vi "Icon Initialization.vi"(7 "LabVIEW Icon in":string, 8 "error in (no error)":errorcluster, 11 "Data in":T1={"Class"={"Ants"=refnum, "Layer"=refnum, "Templates"=refnum, "Icon"=refnum, "Glyph"=refnum, "Settings"=refnum, "Tools"=refnum}, "Ref"={"Add Layer"=refnum, "Remove Layer"=refnum, "Line Text"=[], "Body Text Spec"=refnum, "DNL_Font"=refnum, "glyph path str"=refnum, "templates path str"=refnum, "Arrow Up"=refnum, "Arrow Down"=refnum, "IE VI Ref"=refnum, "Glyphs tree"=refnum, "Templates tree"=refnum, "Layer Icon Text"=refnum, "Layer Template"=refnum, "Clipboard"=refnum, "BW icon in"=refnum, "Color icon in"=refnum, "Layer Clust"=refnum, "Body Text"=refnum, "DNL_Framework Templates"=refnum, "Search Templates"=refnum, "TextMarker"=refnum, "Tab Control"=refnum, "Search Glyphs"=refnum, "Line Color"=refnum, "DNL_Glyphs []"=refnum, "Fill Color"=refnum, "Tools"=refnum, "Glyphs tree"=refnum, "Icon"=refnum, "Preview"=refnum, "Ants"=refnum, "Terminals"=refnum, "menu reference"=refnum, "LayerNames"=[], "GlyphLoadAnimation"=refnum, "TemplateLoadAnimation"=refnum, "refreshGlyphs"=refnum, "refreshTemplates"=refnum}, "Support"={"AntsRect"={"left"=0, "top"=0, "right"=0, "bottom"=0}, "Mouse Move Coords"={"Horizontal"=0, "Vertical"=0}, "Mouse Down Coords"={"Horizontal"=0, "Vertical"=0}, "Temp Coord"={"Horizontal"=0, "Vertical"=0}, "Action"=enum."Default", "Edge Color"=4914962, "Fill Color"=16860, "Mouse Down?"=FALSE, "Draft Mode?"=FALSE, "Temp Icon"=bytes[3102], "CTRL Pressed"=FALSE, "Move Selection?"=FALSE, "AntsRect Orig"={"left"=0, "top"=0, "right"=0, "bottom"=0}, "Text"="", "TM Set?"=FALSE, "Mouse inside icon?"=FALSE, "Tool (old value)"=0, "Pencil Move Color"=0, "Swap Colors?"=FALSE, "Shift pressed?"=FALSE}}) -> (0 "error out":errorcluster, 3 "Data out":T1={"Class"={"Ants"=refnum, "Layer"=refnum, "Templates"=refnum, "Icon"=refnum, "Glyph"=refnum, "Settings"=refnum, "Tools"=refnum}, "Ref"={"Add Layer"=refnum, "Remove Layer"=refnum, "Line Text"=[], "Body Text Spec"=refnum, "DNL_Font"=refnum, "glyph path str"=refnum, "templates path str"=refnum, "Arrow Up"=refnum, "Arrow Down"=refnum, "IE VI Ref"=refnum, "Glyphs tree"=refnum, "Templates tree"=refnum, "Layer Icon Text"=refnum, "Layer Template"=refnum, "Clipboard"=refnum, "BW icon in"=refnum, "Color icon in"=refnum, "Layer Clust"=refnum, "Body Text"=refnum, "DNL_Framework Templates"=refnum, "Search Templates"=refnum, "TextMarker"=refnum, "Tab Control"=refnum, "Search Glyphs"=refnum, "Line Color"=refnum, "DNL_Glyphs []"=refnum, "Fill Color"=refnum, "Tools"=refnum, "Glyphs tree"=refnum, "Icon"=refnum, "Preview"=refnum, "Ants"=refnum, "Terminals"=refnum, "menu reference"=refnum, "LayerNames"=[], "GlyphLoadAnimation"=refnum, "TemplateLoadAnimation"=refnum, "refreshGlyphs"=refnum, "refreshTemplates"=refnum}, "Support"={"AntsRect"={"left"=0, "top"=0, "right"=0, "bottom"=0}, "Mouse Move Coords"={"Horizontal"=0, "Vertical"=0}, "Mouse Down Coords"={"Horizontal"=0, "Vertical"=0}, "Temp Coord"={"Horizontal"=0, "Vertical"=0}, "Action"=enum."Default", "Edge Color"=4914962, "Fill Color"=16860, "Mouse Down?"=FALSE, "Draft Mode?"=FALSE, "Temp Icon"=bytes[3102], "CTRL Pressed"=FALSE, "Move Selection?"=FALSE, "AntsRect Orig"={"left"=0, "top"=0, "right"=0, "bottom"=0}, "Text"="", "TM Set?"=FALSE, "Mouse inside icon?"=FALSE, "Tool (old value)"=0, "Pencil Move Color"=0, "Swap Colors?"=FALSE, "Shift pressed?"=FALSE}})   [LabVIEW 2021]
uses:
  Controls/IE Data.ctl
  Class/Ants/Ants.lvclass
  Class/FakedArray/FakedArray.lvclass
  vi.lib/LabVIEW Icon API/lv_icon/Classes/Icon/Icon.lvclass
  Class/Icon Library/Glyph.lvclass
  Class/Settings/Settings.lvclass
  Class/Tools/Tools Paint.lvclass
  Controls/IE Classes.ctl
  Controls/References Cluster.ctl
  Controls/SupportClass.ctl
  <vilib>/Utility/miscctls.llb/LVPoint32TypeDef.ctl
  Controls/SupportClass_Action.ctl
  vi.lib/LabVIEW Icon API/lv_icon/Controls/IEColor.ctl
  <vilib>/picture/picture.llb/imagedata.ctl
  vi.lib/LabVIEW Icon API/lv_icon/Classes/Layer/Layer.lvclass
  vi.lib/LabVIEW Icon API/LabVIEW Icon API.lvlib
panel:
  in  "Layer":string="Text"
  in  "Template":string="Template"
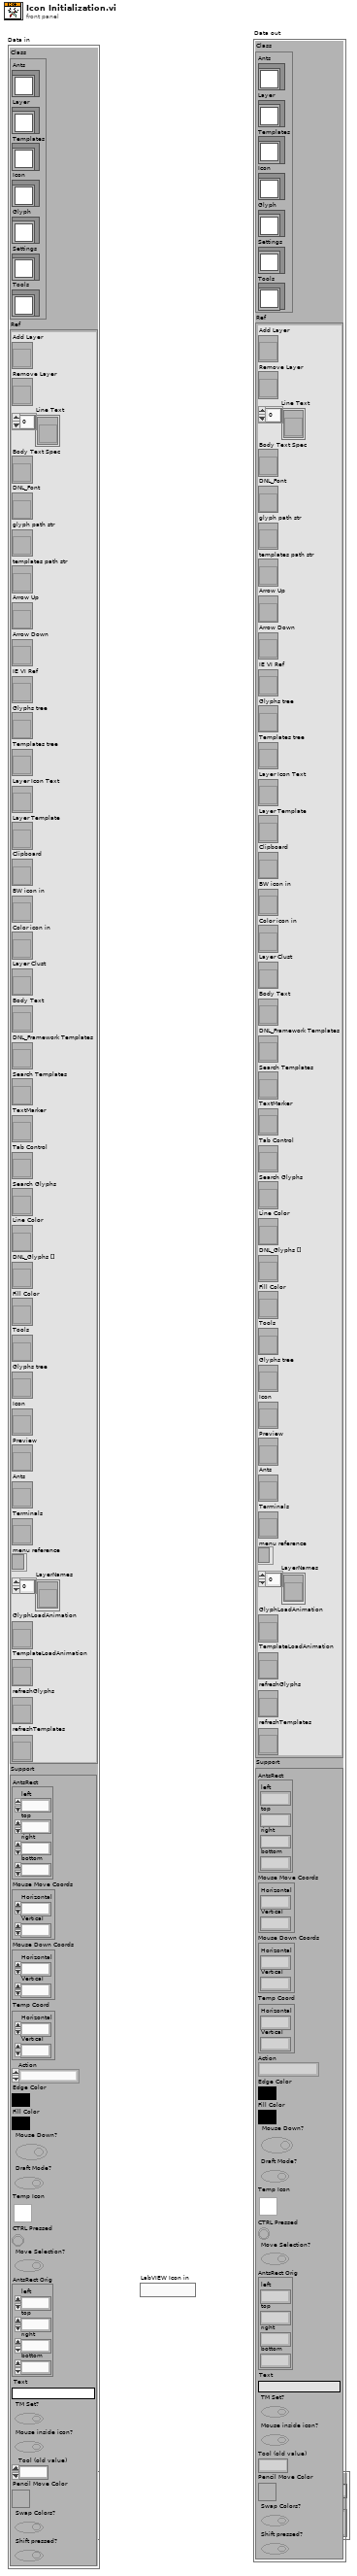
[diagram p1: front panel]
types:
  T1 = typedef "IE Data.ctl" = cluster{"Class":T2, "Ref":T3, "Support":T4}
  T2 = typedef "IE Classes.ctl" = cluster{"Ants":refnum<class "Ants.lvclass">, "Layer":refnum<class "FakedArray.lvclass">, "Templates":refnum<class "FakedArray.lvclass">, "Icon":refnum<class "Icon.lvclass">, "Glyph":refnum<class "Glyph.lvclass">, "Settings":refnum<class "Settings.lvclass">, "Tools":refnum<class "Tools Paint.lvclass">}
  T3 = typedef "References Cluster.ctl" = cluster{"Add Layer":refnum<vi>, "Remove Layer":refnum<vi>, "Line Text":refnum<vi>[], "Body Text Spec":refnum<vi>, "DNL_Font":refnum<vi>, "glyph path str":refnum<vi>, "templates path str":refnum<vi>, "Arrow Up":refnum<vi>, "Arrow Down":refnum<vi>, "IE VI Ref":refnum<vi>, "Glyphs tree":refnum<vi>, "Templates tree":refnum<vi>, "Layer Icon Text":refnum<vi>, "Layer Template":refnum<vi>, "Clipboard":refnum<vi>, "BW icon in":refnum<vi>, "Color icon in":refnum<vi>, "Layer Clust":refnum<vi>, "Body Text":refnum<vi>, "DNL_Framework Templates":refnum<vi>, "Search Templates":refnum<vi>, "TextMarker":refnum<vi>, "Tab Control":refnum<vi>, "Search Glyphs":refnum<vi>, "Line Color":refnum<vi>, "DNL_Glyphs []":refnum<vi>, "Fill Color":refnum<vi>, "Tools":refnum<vi>, "Glyphs tree":refnum<vi>, "Icon":refnum<vi>, "Preview":refnum<vi>, "Ants":refnum<vi>, "Terminals":refnum<vi>, "menu reference":refnum<k9>, "LayerNames":refnum<vi>[], "GlyphLoadAnimation":refnum<vi>, "TemplateLoadAnimation":refnum<vi>, "refreshGlyphs":refnum<vi>, "refreshTemplates":refnum<vi>}
  T4 = typedef "SupportClass.ctl" = cluster{"AntsRect":cluster{"left":i16, "top":i16, "right":i16, "bottom":i16}, "Mouse Move Coords":T5, "Mouse Down Coords":T5, "Temp Coord":T5, "Action":T6, "Edge Color":T7, "Fill Color":T7, "Mouse Down?":bool, "Draft Mode?":bool, "Temp Icon":picture, "CTRL Pressed":bool, "Move Selection?":bool, "AntsRect Orig":cluster{"left":i16, "top":i16, "right":i16, "bottom":i16}, "Text":string, "TM Set?":bool, "Mouse inside icon?":bool, "Tool (old value)":u32, "Pencil Move Color":u32, "Swap Colors?":bool, "Shift pressed?":bool}
  T5 = typedef "LVPoint32TypeDef.ctl" = cluster{"Horizontal":i32, "Vertical":i32}
  T6 = typedef "SupportClass_Action.ctl" = enum16{"Default", "Move Selection", "Glyph Library", "Tool"}
  T7 = typedef "IEColor.ctl" = u32
  T8 = typedef "Who Invoked Icon Editor.ctl" = cluster{"Icon Editor Invoker Type":T9, "App Refnum of Invoker":refnum<vi>, "Qualified Name of Invoker":string, "Path to Invoker":path}
  T9 = typedef "Icon Editor Invoker Type.ctl" = enum32{"Unknown Icon Source", "VI Icon", "Library Icon (any library type)", "Palette icon", "Icon from App Method"}
  T10 = typedef "imagedata.ctl" = cluster{"image type":i32, "image depth":i32, "image":u8[], "mask":u8[], "colors":u32[], "Rectangle":cluster{"left":i16, "top":i16, "right":i16, "bottom":i16}}
  T11 = typedef "LabVIEW Icon Stored Information.ctl" = cluster{"Text Visible?":bool, "Text Opacity":u8, "Templ Visible?":bool, "Templ Opacity":u8, "Relative Path from 1 to 2":path, "Image":picture, "All User Layers":refnum<class "Layer.lvclass">[], "Body Text":T12}
  T12 = typedef "BodyText.ctl" = cluster{"Line 1 text":string, "Line 2 text":string, "Line 3 text":string, "Line 4 text":string, "Line 1 color":u32, "Line 2 color":u32, "Line 3 color":u32, "Line 4 color":u32, "Body Text Spec":cluster{"Font":T13, "Alignment":T14, "Size":u8}, "Center text vertically":bool, "Capitalize Text":bool}
  T13 = typedef "Font.ctl" = string
  T14 = typedef "Alignment.ctl" = u16
  T15 = cluster{"image type":i32, "image depth":i32, "image":u8[], "mask":u8[], "colors":u32[], "Rectangle":cluster{"left":i16, "top":i16, "right":i16, "bottom":i16}}
  T16 = typedef "Font Size.ctl" = u8
  T17 = cluster{"Line 1 text":string, "Line 2 text":string, "Line 3 text":string, "Line 4 text":string, "Line 1 color":u32, "Line 2 color":u32, "Line 3 color":u32, "Line 4 color":u32, "Body Text Spec":cluster{"DNL_Font":T13, "Alignment":T14, "Size":T16}, "Center text vertically":bool, "Capitalize Text":bool}
  T18 = typedef "Layer.ctl" = cluster{"LayerIcon":picture, "LayerName":string, "Opacity":u8, "Visibility?":bool}
  T19 = typedef "Graphic.ctl" = cluster{"Rectangle":cluster{"left":i16, "top":i16, "right":i16, "bottom":i16}, "Path":path, "Image":picture, "Filter":string, "FileName":string}
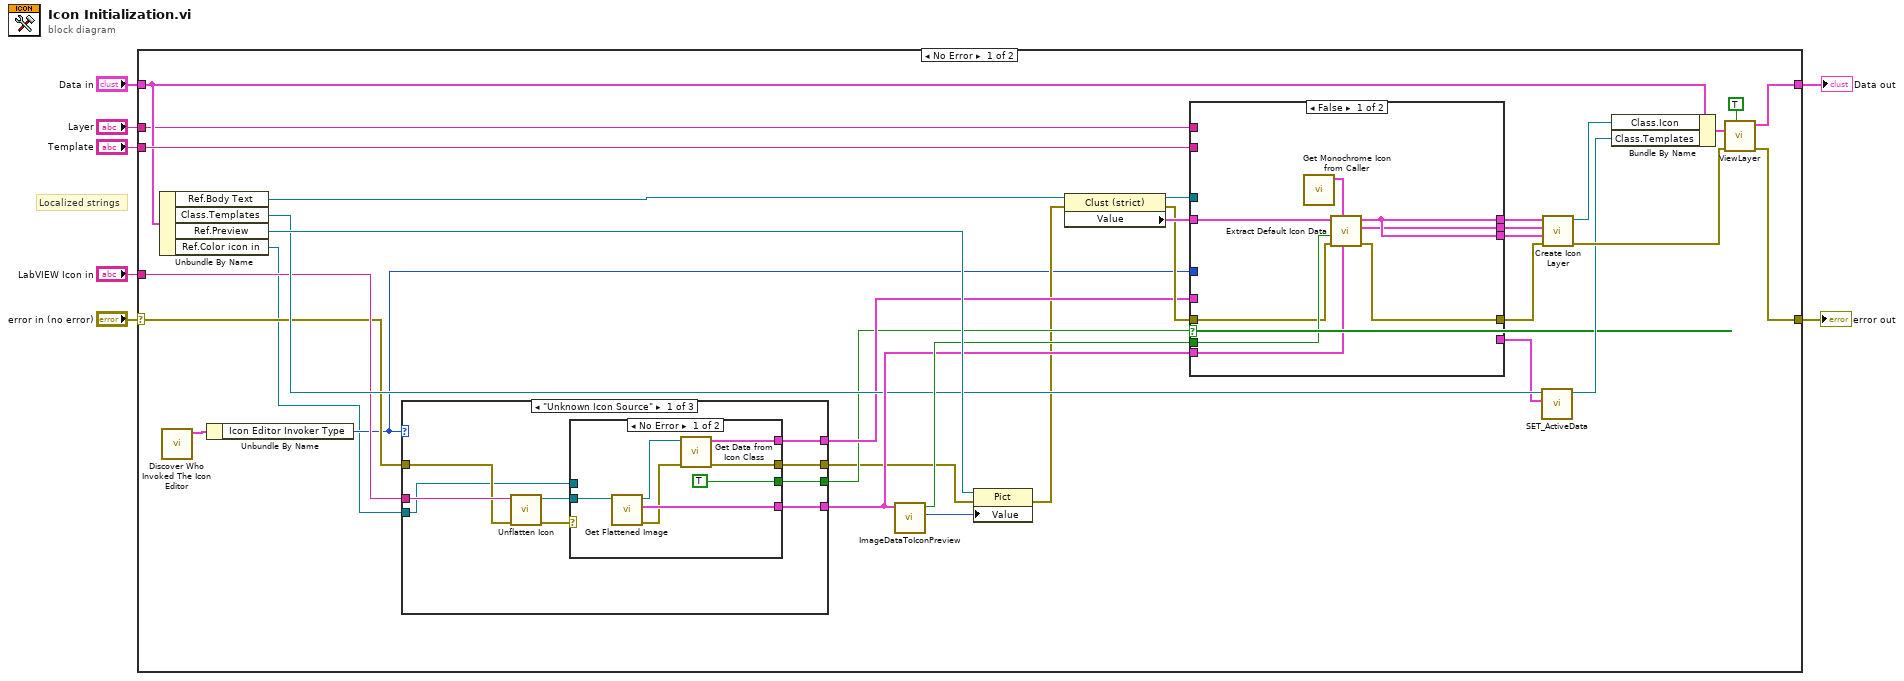
[diagram p0: block diagram]
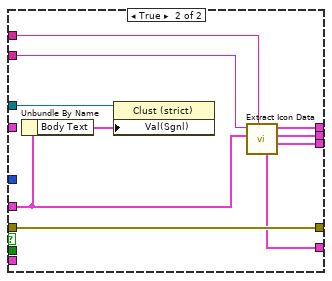
[diagram p2: hidden frame]
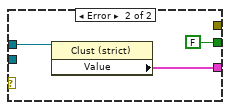
[diagram p3: hidden frame]
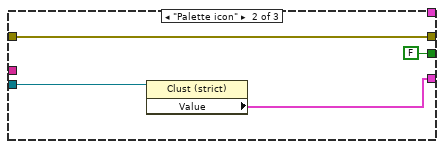
[diagram p4: hidden frame]
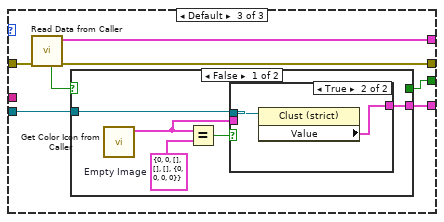
[diagram p5: hidden frame]
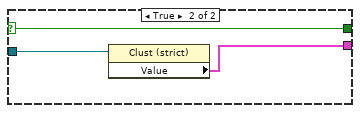
[diagram p7: hidden frame]
diagram:
  # "Localized strings"
  n1 = case shown="No Error" "error in (no error)" {
    selector: "error in (no error)" -> [w13 w101]
    tunnel: [w35 w101] -> w6
    tunnel: "Template" -> [w40 _]
    tunnel: "Data in" -> [w33 w100]
    tunnel: [w34 w100] -> w3
    tunnel: "Layer" -> [w24 _]
    tunnel: "LabVIEW Icon in" -> [w22 _]
    frame No Error {
      n2 = Unbundle By Name(w33) -> ("Ref.Body Text"=w28:refnum<vi>, "Class.Templates"=w26:refnum<class "FakedArray.lvclass">, "Ref.Preview"=w32:refnum<vi>, "Ref.Color icon in"=w8:refnum<vi>)
      n3 = call <resource>:"Discover Who Invoked The Icon Editor.vi"() -> ("Who Invoked The Icon Editor?"=w23:T8)  [unwired: 11 out]
      n4 = Unbundle By Name(w23) -> ("Icon Editor Invoker Type"=w9:T9)
      n5 = case shown="\"Unknown Icon Source\"" w9 {
        tunnel: [w67 w78 w84] -> w29
        tunnel: w22 -> [w64 _ _]
        tunnel: [w65 _ w88] -> w15
        tunnel: w13 -> [w63 w81 w87]
        tunnel: [w66 w81 w86] -> w12
        tunnel: [w60 FALSE ("Valid?") w82] -> w14
        tunnel: w8 -> [w59 w79 w85]
        frame "Unknown Icon Source" {
          n6 = call "Unflatten Icon.vi"("Error In"=w63, "String"=w64) -> ("Error Out"=w61:errorcluster, "Layers"=w62:refnum<class "Icon.lvclass">)  [unwired: 8 in]
          n7 = case shown="No Error" w61 {
            tunnel: [w74 w76] -> w67
            tunnel: [w72 _] -> w66
            tunnel: [w70 _] -> w65
            tunnel: w62 -> [w69 _]
            tunnel: [TRUE ("Valid?") FALSE ("Valid?")] -> w60
            tunnel: w59 -> [_ w77]
            frame No Error {
              n8 = call "Get Flattened Image.vi"("lv_icon.lvlib:Icon.lvclass in"=w69) -> ("error out"=w73:errorcluster, "Color Image"=w74:T10, "lv_icon.lvlib:Icon.lvclass out"=w71:refnum<class "Icon.lvclass">)  [unwired: 7 in, 1 out]
              n9 = call "Get Data from Icon Class.vi"("error in (no error)"=w73, "Icon in"=w71) -> ("error out"=w72:errorcluster, "Icon data"=w70:T11)  [unwired: 6 in, 2 out]
            }
            frame Error {
              n10 = property class="Clust (strict)"(reference=w77) -> ("Value"=w76:T15)  [unwired: 1 in, 2 out]
            }
          }
        }
        frame "Palette icon" {
          n11 = property class="Clust (strict)"(reference=w79) -> ("Value"=w78:T15)  [unwired: 1 in, 2 out]
        }
        frame Default {
          n12 = call "Read Data from Caller.vi"("error in (no error)"=w87) -> ("error out"=w86:errorcluster, "data"=w88:T11, "Valid?"=w83:bool)  [unwired: 2 in, 6 out]
          n13 = case shown="False" w83 {
            selector: w83 -> [_ w99]
            tunnel: w85 -> [w91 w98]
            tunnel: [w89 w97] -> w84
            tunnel: [_ w99] -> w82
            frame False {
              w93 = T10 {"image type"=0, "image depth"=0, "image"=[], "mask"=[], "colors"=[], "Rectangle"={"left"=0, "top"=0, "right"=0, "bottom"=0}}  # Empty Image
              n14 = call "Get Color Icon from Caller.vi"() -> ("color"=w90:T10)  [unwired: 11 in]
              n15 = Equal?(x=w90, y=w93) -> (x = y?=w92:bool)
              n16 = case shown="True" w92 {
                tunnel: w91 -> [_ w96]
                tunnel: w90 -> [w94 _]
                tunnel: [w94 w95] -> w89
                frame False {
                }
                frame True {
                  n17 = property class="Clust (strict)"(reference=w96) -> ("Value"=w95:T15)  [unwired: 1 in, 2 out]
                }
              }
            }
            frame True {
              n18 = property class="Clust (strict)"(reference=w98) -> ("Value"=w97:T15)  [unwired: 1 in, 2 out]
            }
          }
        }
      }
      n19 = call "ImageDataToIconPreview.vi"("Image data in"=w29) -> ("Icon"=w31:picture, "Is default icon?"=w30:bool)  [unwired: 9 in]
      n20 = property class="Pict"(reference=w32, error in=w12, "Value"=w31) -> (error out=w11:errorcluster)  [unwired: 1 out]
      n21 = property class="Clust (strict)"(reference=w28, error in=w11) -> (reference out=w10:refnum<vi>, error out=w18:errorcluster, "Value"=w19:T17)
      n22 = case shown="False" w14 {
        tunnel: w15 -> [_ w50]
        tunnel: w18 -> [w45 w55]
        tunnel: w40 -> [_ w58]
        tunnel: [w44 w57] -> w21
        tunnel: [w48 w55] -> w20
        tunnel: [w44 w56] -> w17
        tunnel: w30 -> [w47 _]
        tunnel: w29 -> [w43 _]
        tunnel: w19 -> [w46 _]
        tunnel: [_ w51] -> w25
        tunnel: [w41 w54] -> w16
        tunnel: w24 -> [_ w53]
        tunnel: w10 -> [_ w52]
        tunnel: w9 -> [_ _]
        frame False {
          n23 = call "Get Monochrome Icon from Caller.vi"() -> ("monochrome"=w42:T10)  [unwired: 11 in]
          n24 = call "Extract Default Icon Data.vi"("Color Icon"=w43, "BW Icon"=w42, "error in (no error)"=w45, "New VI template? (F)"=w47, "Body text"=w46) -> ("error out"=w48:errorcluster, "VI Icon Data out"=w41:T11, "Default Icon Template data"=w44:T18)  [unwired: 4 in]
        }
        frame True {
          n25 = Unbundle By Name(w50) -> ("Body Text"=w49:T12)
          n26 = property class="Clust (strict)"(reference=w52, "Val(Sgnl)"=w49) -> ()  [unwired: 1 in, 2 out]
          n27 = call "Extract Icon Data.vi"("Text layer name"=w53, "Icon data in"=w50, "Template layer name"=w58) -> ("Template data"=w57:T18, "Icon data out"=w54:T11, "Text data"=w56:T18, "Active template (faked Array)"=w51:T19)  [unwired: 5 in]
        }
      }
      n28 = call-dynamic "SET_ActiveData.vi"("Active Data"=w25, "FakedArray.lvclass in"=w26) -> ("FakedArray.lvclass out"=w27:refnum<class "FakedArray.lvclass">)  [unwired: 1 in, 8 out]
      n29 = call "Create Icon Layer.vi"("error in (no error)"=w20, "Template data"=w21, "Icon data"=w16, "Text data"=w17) -> ("error out"=w37:errorcluster, "Icon out"=w39:refnum<class "Icon.lvclass">)  [unwired: 6 in]
      n30 = Bundle By Name(cluster=w33, "Class.Icon"=w39, "Class.Templates"=w27) -> (w36:T1)
      n31 = call "ViewLayer.vi"("Add to Undo?"=TRUE, "error in (no error)"=w37, "Data in"=w36) -> ("error out"=w35:errorcluster, "Data out"=w34:T1)  [unwired: 1 in, 6 out]
    }
    frame Error {
    }
  }
  "error out" <- w6
  "Data out" <- w3
